vi "Write GFOC old2.vi"(8 "error in (no error)":errorcluster, 10 "Opt_Selector.lvclass":refnum<class "Opt_Selector.lvclass">, 11 "Instrument in":refnum<class "Instrument.lvclass">) -> (0 "error out":errorcluster, 3 "Instrument out":refnum<class "Instrument.lvclass">)   [LabVIEW 2018]
uses:
  Instrument.lvclass
  C:/Users/observer/Desktop/Sparc4GUI/SPARC4_GUI/Server/Server.lvclass
  Device/Optics/Opt_Selector/Opt_Selector.lvclass
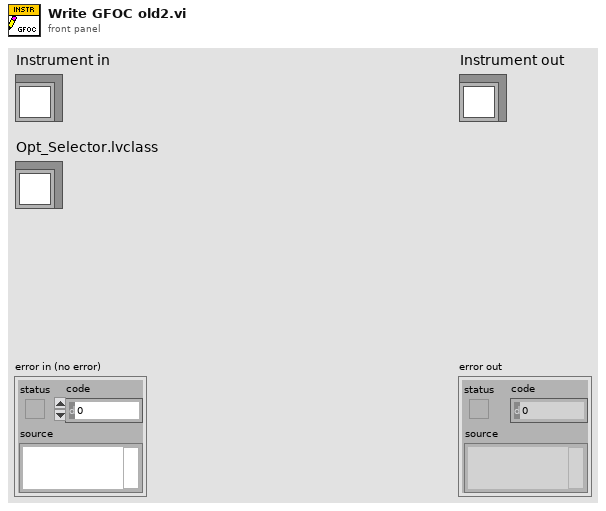
[diagram p1: front panel]
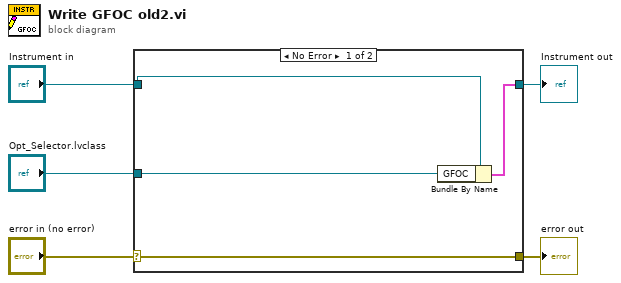
[diagram p0: block diagram]
diagram:
  n1 = case shown="No Error" "error in (no error)" {
    selector: "error in (no error)" -> [w9 w10]
    tunnel: [w9 w10] -> w4
    tunnel: [w7 w11] -> w2
    tunnel: "Instrument in" -> [w8 w11]
    tunnel: "Opt_Selector.lvclass" -> [w6 _]
    frame No Error {
      n2 = Bundle By Name(cluster=w8, "GFOC"=w6) -> (w7:cluster{})
    }
    frame Error {
    }
  }
  "error out" <- w4
  "Instrument out" <- w2
